vi "gyro -- launch async sweeper.vi"(11 "sweeper event pair":T1) -> (2 "reference out":refnum<vi>, 3 "sweeper event pair OUT":T1)   [LabVIEW 2018]
uses:
  server talkback message type.ctl
  server talkto message type.ctl
  server talk-to-back pair.ctl
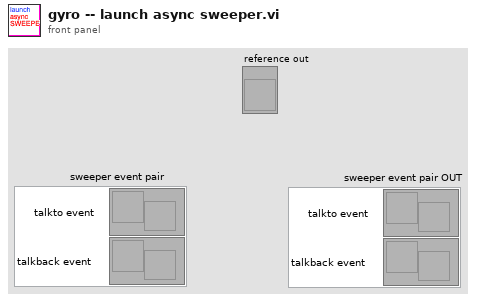
[diagram p1: front panel]
types:
  T1 = typedef "server talk-to-back pair.ctl" = cluster{"talkback event":refnum<user-event>, "talkto event":refnum<user-event>}
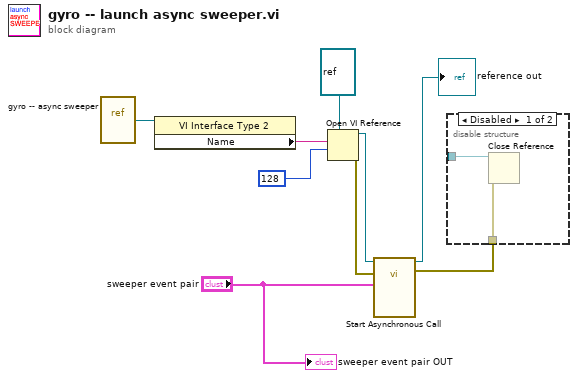
[diagram p0: block diagram]
diagram:
  n1 = vi-ref "gyro -- async sweeper.vi"() -> (w7:refnum<vi>)
  n2 = property class="VI Interface Type 2"(reference=w7) -> ("Name"=w6:string)  [unwired: 1 in, 2 out]
  n3 = Open VI Reference(type specifier VI Refnum (for type only)=refnum<vi> refnum, vi path=w6, options=128) -> (vi reference=w8:refnum<vi>, error out=w3:errorcluster)  [unwired: 3 in]
  n4 = call-by-ref "Start Asynchronous Call"(reference=w8, error in=w3, "pll event pair"="sweeper event pair") -> (reference out=→"reference out":refnum<vi>, error out=w4:errorcluster)  [unwired: 11 in]
  n5 = disable-structure shown="Disabled" {
    disable-tunnel: w4 -> [w11 _]
    disable-tunnel: _ -> [w10 _]
    frame Disabled {
      n6 = Close Reference(reference=w10, error in (no error)=w11) -> ()  [unwired: 1 out]
    }
    frame Enabled {
    }
  }
  "sweeper event pair OUT" <- "sweeper event pair"
